vi "WriteU16.vi"(1 "U16":u16, 2 "FIFO":refnum<k21>="DisplacementTxFIFO") -> ()   [LabVIEW 2016, in "FPGAFIFO.lvlib"]
uses:
  FPGAFIFO.lvlib
  <vilib>/rvi/DataTransferAndStorage/Container/Common/niFpgaContainerExecOnDevCompGetState.vi
  <vilib>/rvi/Emulation/niFpgaEmulationIsFPGAContextNoSignature.vi
  <vilib>/rvi/Emulation/niFpgaSctlEmulationGetInTimedLoop.vi
  <vilib>/rvi/errors/niFpgaSetErrorForExecOnDevCompSimple.vi
  <vilib>/rvi/eio/common/nirviEmuReportErrorAndStop.vi
  <vilib>/rvi/DataTransferAndStorage/Container/Common/niFpgaContainerGetUniqueNameForEmu.vi
  <vilib>/rvi/FIFO/Fifo_Resource/nirvififoEmulationSetSize.vi
  <vilib>/rvi/FIFO/Fifo_Resource/nirviFifoEmulationQueueMgr.vi
  <instcachedir>/0/nirviFifoEmulationQueueMgr_E5CAEC123FF24DC58D834DCA3CDAA9B5.lvgen/nirviFifoEmulationQueueMgr_E5CAEC123FF24DC58D834DCA3CDAA9B5_009.vi
  <vilib>/rvi/FIFO/Fifo_Resource/nirvififoEmulationDetermineInputValidOut.vi
  <vilib>/rvi/FIFO/Fifo_Resource/nirvififoEmulationCreateLock.vi
  <vilib>/rvi/Emulation/niFpgaProcessEmulError.vi
  <vilib>/rvi/FIFO/Fifo_Resource/nirvififoEmulationObtainLock.vi
  <vilib>/rvi/FIFO/Fifo_Resource/nirvififoEmulationReleaseLock.vi
  <vilib>/rvi/occurrence/nirviWaitOnOccurrenceBase.vi
  <vilib>/rvi/errors/nirviReportUnexpectedCaseInternalError.vi
  <vilib>/rvi/errors/nirviReportUnexpectedCaseInternalError (U32).vi
  <vilib>/Utility/error.llb/Clear Errors.vi
  <vilib>/rvi/interface/RandomDataEmulation/niFpgaRandomDataHandleErrors.vi
  <vilib>/rvi/DataTransferAndStorage/Container/XNode/niFpgaContainer.xnode
  <vilib>/rvi/FIFO/Fifo_Resource/niFpgaFifoEmulationRefIn.vi
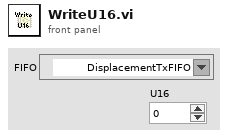
[diagram p1: front panel]
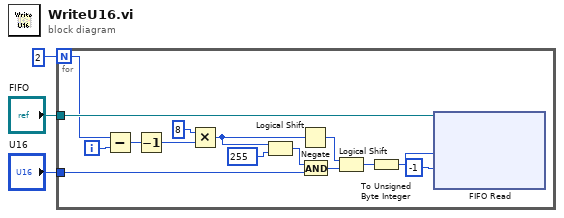
[diagram p0: block diagram]
diagram:
  n1 = for {
    N: 2 -> [w16]
    tunnel: "FIFO" -> [w18]
    tunnel: "U16" -> [w9]
    i -> [w15]
    n2 = Subtract(x=w16, y=w15) -> (x-y=w13:i32)
    n3 = Decrement(x=w13) -> (x-1=w12:i32)
    n4 = Multiply(x=8 ("y"), y=w12) -> (x*y=w7:i32)
    n5 = Logical Shift(y=w7, x=u16 255) -> (x << y=w10:u16)
    n6 = Negate(x=w7) -> (-x=w6:i32)
    n7 = And(x=w10, y=w9) -> (x .and. y?=w8:u16)
    n8 = Logical Shift(y=w6, x=w8) -> (x << y=w5:u16)
    n9 = To Unsigned Byte Integer(number=w5) -> (unsigned 8bit integer=w4:u8)
    n10 = xnode "FIFO Read"("Element"=w4, "Timeout"=-1, "FIFO In"=w18) -> ()  [unwired: 2 out]
  }
